vi "Aktualizuj skale przebiegow.vi"(7 "Przebiegi":waveform(dbl)[](array[waveform]), 8 "error in (no error)":errorcluster, 9 "PlotIdx":i32, 11 "WaveformGraph in":refnum<vi>) -> (0 "error out":errorcluster)   [LabVIEW 2014]
doc: "Aktualizuje widoczność skal przebiegów na wykresie\njeżeli nie ma żadnego widocznego przebiegu\nw danej skali - wyłącza widoczność skali\njeżeli jest co najmniej jeden widoczny przebieg włącza"
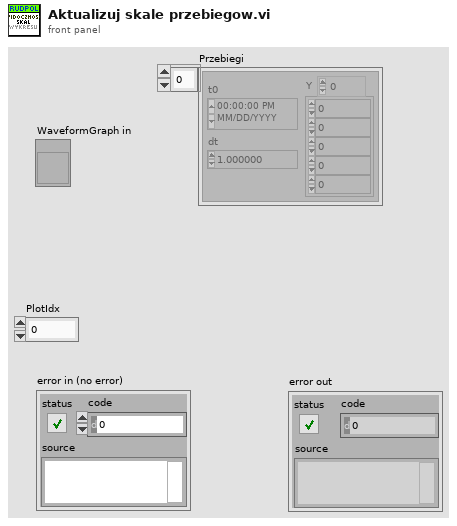
[diagram p1: front panel]
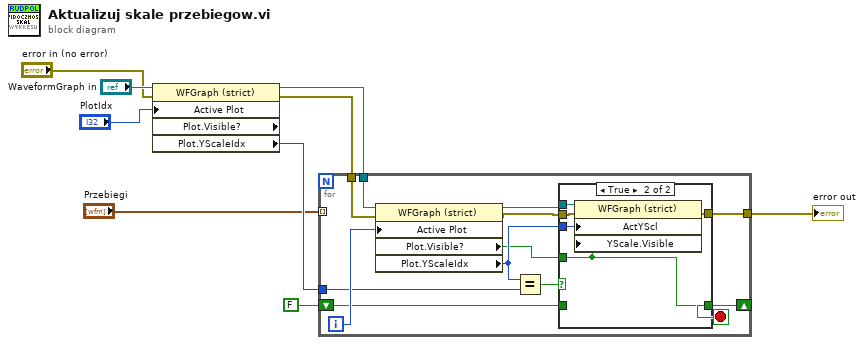
[diagram p0: block diagram]
diagram:
  n1 = property on="Property Node" class="WFGraph (strict)" props=["Active Plot", "Plot", "Visible?", "Plot", "YScaleIdx"](reference="WaveformGraph in", error in="error in (no error)", "Active Plot"="PlotIdx") -> (reference out=w3:refnum<vi>, error out=w2:errorcluster, "Plot.YScaleIdx"=w8:u32)  [unwired: 1 out]
  n2 = for {
    tunnel: "Przebiegi" -> [_] mode=indexing
    tunnel: w8 -> [w20]
    shift-right: [w16] -> _
    shift-left: FALSE -> [w17]
    tunnel: w3 -> [w15]
    tunnel: w2 -> [w12]
    tunnel: [w11] -> w1
    i -> [w21]
    stop <- w16 stop-if-true
    n3 = property on="Property Node" class="WFGraph (strict)"(reference=w15, error in=w12, "Active Plot"=w21) -> (reference out=w14:refnum<vi>, error out=w13:errorcluster, "Plot.Visible?"=w10:bool, "Plot.YScaleIdx"=w19:u32)
    n4 = Equal?(x=w19, y=w20) -> (x = y?=w18:bool)
    n5 = case shown="True" w18 {
      tunnel: w19 -> [_ w28]
      tunnel: w17 -> [w23 _]
      tunnel: [w23 w27] -> w16
      tunnel: w10 -> [_ w27]
      tunnel: w14 -> [_ w26]
      tunnel: w13 -> [w22 w25]
      tunnel: [w22 w24] -> w11
      frame False {
      }
      frame True {
        n6 = property on="Property Node" class="WFGraph (strict)"(reference=w26, error in=w25, "ActYScl"=w28, "YScale.Visible"=w27) -> (error out=w24:errorcluster)  [unwired: 1 out]
      }
    }
  }
  "error out" <- w1
